vi "create engine.vi"(8 "error in":errorcluster) -> (0 "error out":errorcluster, 3 "engine":u64)   [LabVIEW 2016, in "async tls dl.lvlib"]
uses:
  async tls dl.lvlib
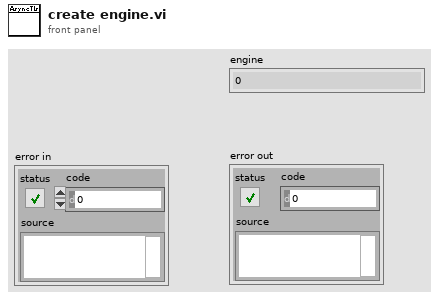
[diagram p1: front panel]
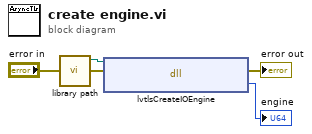
[diagram p0: block diagram]
diagram:
  n1 = call "library path.vi"() -> ("path"=w1:path)  [unwired: 11 in]
  n2 = dll-call lib="C:/Users/IEUser/Desktop/libasynclvtls/lvasynctls.dll" fn="lvtlsCreateIOEngine"(path in=w1, error in="error in") -> (error out=→"error out":errorcluster, "engine"=→"engine":u64)  [unwired: 1 in, 1 out]
